vi "PIDTEMPtest5.vi"() -> ()   [LabVIEW 2015]
uses:
  <vilib>/DAQmx/write.llb/DAQmx Write (Digital 1D Bool NChan 1Samp 1Line).vi
  <vilib>/DAQmx/write.llb/DAQmx Write (Digital Bool 1Line 1Point).vi
  <vilib>/DAQmx/read.llb/DAQmx Read (Analog DBL 1Chan 1Samp).vi
  <vilib>/DAQmx/miscellaneous.llb/DAQmx Fill In Error Info.vi
  <vilib>/addons/control/pid/NI_PID_autopid.lvlib
panel:
  in  "Heater On/Off":bool
  in  "Manual Control":bool
  in  "stop 2":bool
  out "ms to wait":dbl
  out "Control Value":dbl
  in  "setpoint in C":dbl format="%.2f"
  in  "reinitialize? (F)":bool
  in  "autotune? (F)":bool
  out "PID gains out":T1={"proportional gain (Kc)"=1.0, "integral time (Ti, min)"=0.01, "derivative time (Td, min)"=0.0} {"derivative time (Td, min)" format="%.3f"; "integral time (Ti, min)" format="%.3f"; "proportional gain (Kc)" format="%.3f"}
  in  "PID gains":T1={"proportional gain (Kc)"=1.0, "integral time (Ti, min)"=0.01, "derivative time (Td, min)"=0.0} {"derivative time (Td, min)" format="%.3f"; "integral time (Ti, min)" format="%.3f"; "proportional gain (Kc)" format="%.3f"}
  in  "autotuning parameters":T2={"controller type"=1, "relay cycles"=3, "relay amplitude"=1.0, "control specification"=2, "PV noise level"=0.1} {"PV noise level" format="%.2f"; "control specification" items=["normal", "fast", "slow"]; "relay amplitude" format="%.2f"; "controller type" items=["PID", "PI", "P"]}
  in  "stop":bool
  out "Temp":dbl
  out "Temp Chart 2":dbl(graph)
  out "Temp Chart":dbl(graph)
  out "Temp(C)":dbl(slide) scale=-10.0..100.0
  out "Temperature (Celcius)":dbl format="%#.1g"
  out "Voltage Reading(Temp)":dbl format="%#_13g"
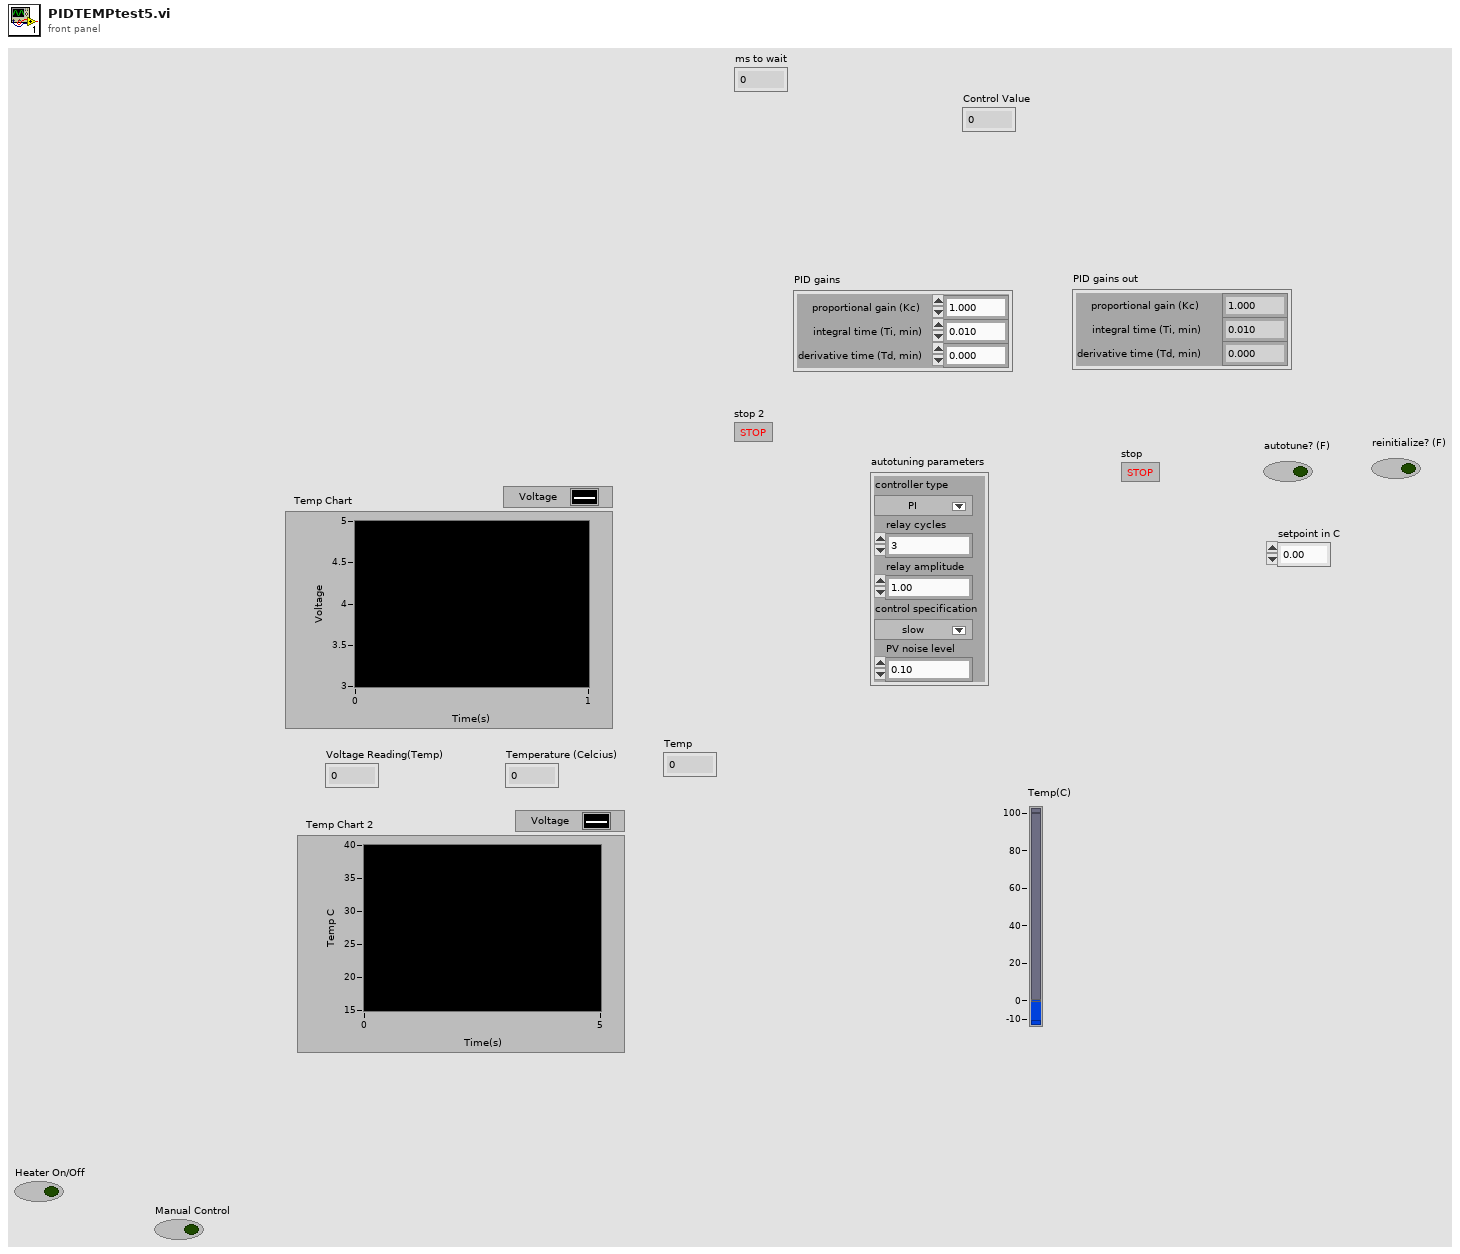
[diagram p1: front panel]
types:
  T1 = cluster{"proportional gain (Kc)":dbl, "integral time (Ti, min)":dbl, "derivative time (Td, min)":dbl}
  T2 = cluster{"controller type":u16, "relay cycles":i32, "relay amplitude":dbl, "control specification":u16, "PV noise level":dbl}
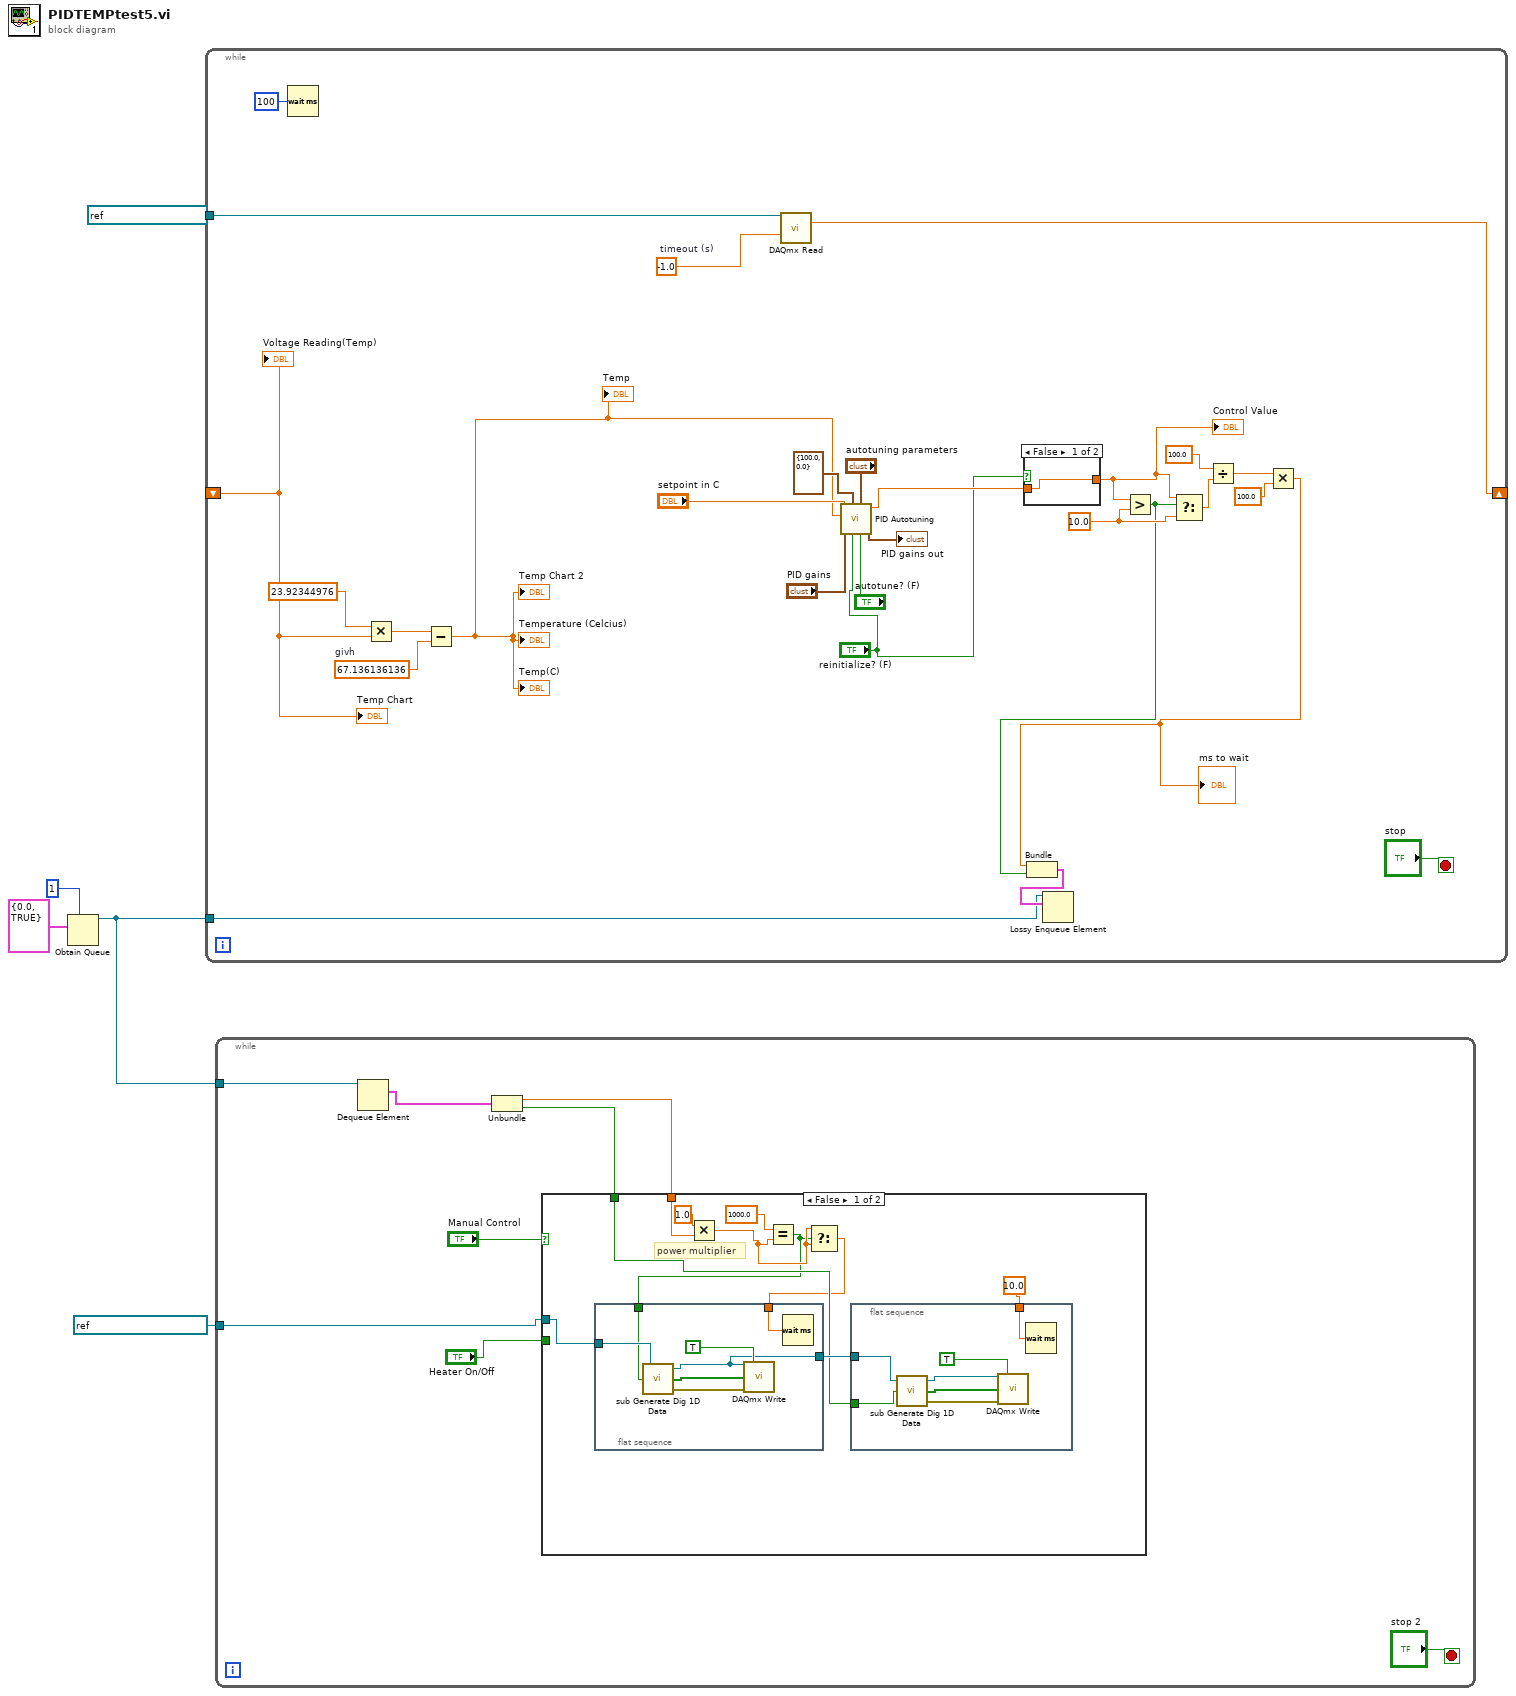
[diagram p0: block diagram]
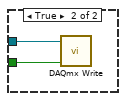
[diagram p2: hidden frame]
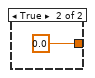
[diagram p3: hidden frame]
diagram:
  n1 = Obtain Queue(max queue size (-1, unlimited)=1, element data type=cluster{dbl, bool} {0.0, TRUE}) -> (queue out=w3:refnum<queue>)  [unwired: 3 in, 2 out]
  n2 = while {
    tunnel: refnum<k21> "MyVoltageTask_0" -> [w29]
    shift-right: [w11] -> _
    shift-left: _ -> [w12]
    tunnel: w3 -> [w6]
    stop <- "stop" stop-if-true
    w14 = 10.0 ("f")
    w30 = 67.136136136  # givh
    w33 = -1.0  # timeout (s)
    n3 = Wait (ms)(milliseconds to wait=u32 100) -> ()  [unwired: 1 out]
    n4 = Multiply(x=23.92344976, y=w12) -> (x*y=w31:dbl)
    n5 = Subtract(x=w31, y=w30) -> (x-y=w10:dbl)
    "Temperature (Celcius)" <- w10
    "Temp(C)" <- w10
    "Temp Chart 2" <- w10
    "Temp" <- w10
    n6 = call-poly <vilib>:"DAQmx Read.vi"("task/channels in"=w29, "timeout"=w33) -> ("data"=w11:dbl)  [unwired: 11 in, 2 out]
    n7 = call <vilib>:"PID Autotuning.vi"("autotune? (F)"="autotune? (F)", "autotuning parameters"="autotuning parameters", "reinitialize? (F)"="reinitialize? (F)", "output range"=cluster{"output high":dbl, "output low":dbl} {"output high"=100.0, "output low"=0.0}, "PID gains"="PID gains", "process variable"=w10, "setpoint"="setpoint in C") -> ("PID gains out"=→"PID gains out":T1, "output"=w22:dbl)  [unwired: 1 in, 2 out]
    n8 = case shown="False" "reinitialize? (F)" {
      tunnel: [w34 0.0] -> w15
      tunnel: w22 -> [w34 _]
      frame False {
      }
      frame True {
      }
    }
    "Control Value" <- w15
    n9 = Greater?(x=w15, y=w14) -> (0:w8:bool)
    n10 = Select(t=w15, s=w8, f=w14) -> (s? t:f=w16:dbl)
    n11 = Divide(x=100.0, y=w16) -> (x/y=w18:dbl)
    n12 = Multiply(x=w18, y=100.0) -> (x*y=w9:dbl)
    "ms to wait" <- w9
    n13 = Bundle(w9, w8) -> (w7:cluster{dbl, bool})  [unwired: 1 in]
    n14 = Lossy Enqueue Element(queue=w6, element=w7) -> ()  [unwired: 1 in, 4 out]
    "Voltage Reading(Temp)" <- w12
    "Temp Chart" <- w12
  }
  n15 = while {
    tunnel: w3 -> [w43]
    tunnel: refnum<k21> "MyDigitalOutTask_2" -> [w39]
    stop <- "stop 2" stop-if-true
    n16 = Dequeue Element(queue=w43) -> (element=w38:cluster{dbl, bool})  [unwired: 2 in, 3 out]
    n17 = Unbundle(w38) -> (w37:dbl, w36:bool)
    n18 = case shown="False" "Manual Control" {
      tunnel: w39 -> [w52 w69]
      tunnel: "Heater On/Off" -> [_ w68]
      tunnel: w37 -> [w51 _]
      tunnel: w36 -> [w49 _]
      frame False {
        # "power multiplier"
        n19 = flat-sequence {
          tunnel: w52 -> [w64]
          tunnel: [w63] -> w53
          tunnel: w46 -> [w62]
          tunnel: w45 -> [w61]
          frame #0 {
            n20 = call <vilib>:"sub Generate Dig 1D Data.vi"("initial value"=w62, "task in"=w64) -> ("error out"=w66:errorcluster, "Data"=w67:bool[], "task out"=w63:refnum<k21>)  [unwired: 1 in]
            n21 = call-poly <vilib>:"DAQmx Write.vi"("task/channels in"=w63, "auto start"=TRUE, "data"=w67, "error in"=w66) -> ()  [unwired: 9 in, 3 out]
            n22 = Wait (ms)(milliseconds to wait=w61) -> ()  [unwired: 1 out]
          }
        }
        n23 = Multiply(x=1.0, y=w51) -> (x*y=w47:dbl)
        n24 = Equal?(x=1000.0, y=w47) -> (x = y?=w46:bool)
        n25 = Select(t=w47, s=w46, f=w47) -> (s? t:f=w45:dbl)
        n26 = flat-sequence {
          tunnel: w53 -> [w56]
          tunnel: 10.0 -> [w55]
          tunnel: w49 -> [w54]
          frame #0 {
            n27 = call <vilib>:"sub Generate Dig 1D Data.vi"("initial value"=w54, "task in"=w56) -> ("error out"=w59:errorcluster, "Data"=w57:bool[], "task out"=w58:refnum<k21>)  [unwired: 1 in]
            n28 = call-poly <vilib>:"DAQmx Write.vi"("task/channels in"=w58, "auto start"=TRUE, "data"=w57, "error in"=w59) -> ()  [unwired: 9 in, 3 out]
            n29 = Wait (ms)(milliseconds to wait=w55) -> ()  [unwired: 1 out]
          }
        }
      }
      frame True {
        n30 = call-poly <vilib>:"DAQmx Write.vi"("task/channels in"=w69, "data"=w68) -> ()  [unwired: 11 in, 3 out]
      }
    }
  }
